vi "FTW-DevUtil-CLFNPrototypes.vi"(0 "VI Ref":refnum<vi>, 11 "error in":errorcluster) -> (4 "VI Ref out":refnum<vi>, 6 "CLFNs":T1[](array[typedef]), 15 "error out":errorcluster)   [LabVIEW 2015]
uses:
  FTW-DevUtil-CLFNPrototype.ctl
panel:
  # "Inputs"
  # "Outputs"
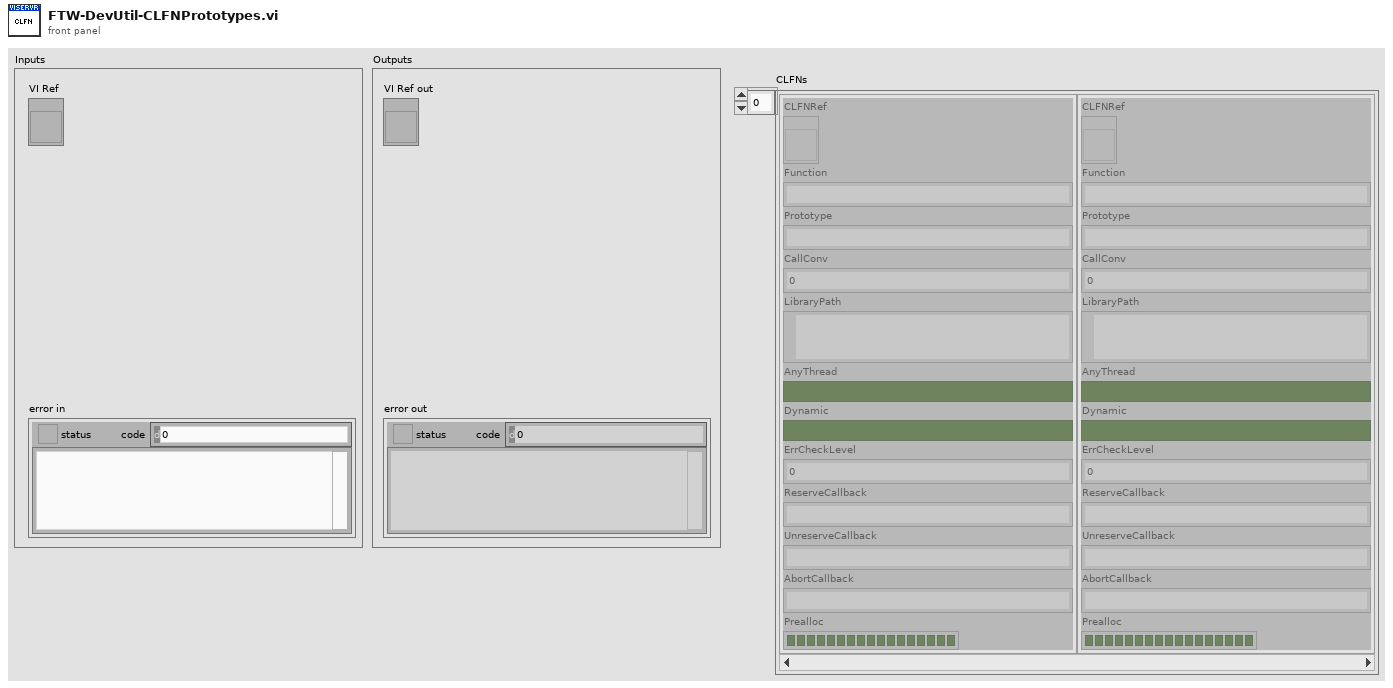
[diagram p1: front panel]
types:
  T1 = typedef "FTW-DevUtil-CLFNPrototype.ctl" = cluster{"CLFNRef":refnum<vi>, "Function":string, "Prototype":string, "CallConv":u32, "LibraryPath":path, "Debug":bool, "Debug":bool, "ErrCheckLevel":u32, "ReserveCallback":string, "UnreserveCallback":string, "AbortCallback":string, "Prealloc":bool[]}
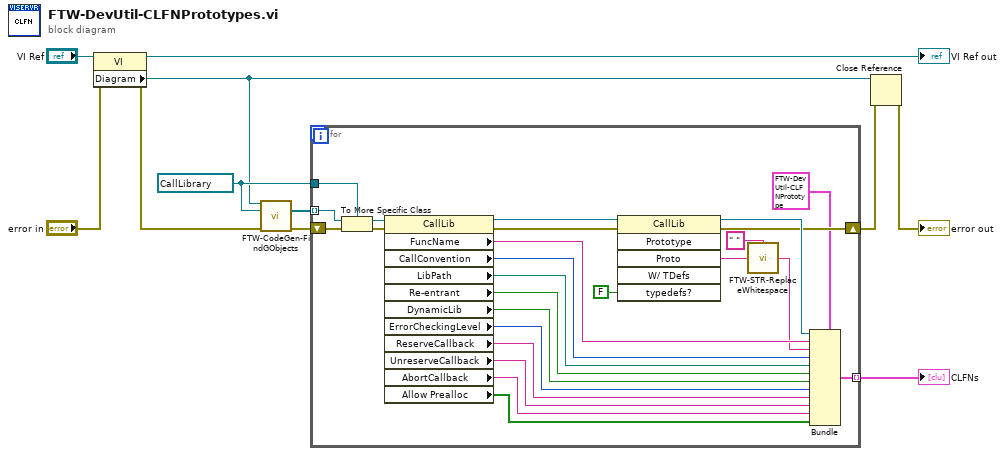
[diagram p0: block diagram]
diagram:
  w9 = refnum<vi> refnum ("GObject")
  n1 = property class="VI"(reference="VI Ref", error in="error in") -> (reference out=→"VI Ref out":refnum<vi>, error out=w4:errorcluster, "Diagram"=w3:refnum<vi>)
  n2 = call "FTW-CodeGen-FindGObjects.vi"("GObject to Traverse"=w3, "Class Type Reference"=w9, "error in"=w4) -> ("GObject Instances"=w11:refnum<vi>[], "error out"=w10:errorcluster)  [unwired: 11 in]
  n3 = for {
    tunnel: w11 -> [w36] mode=indexing
    tunnel: w9 -> [w35]
    tunnel: [w32] -> w7 mode=indexing
    shift-right: [w13] -> w2
    shift-left: w10 -> [w34]
    n4 = To More Specific Class(target class=w35, reference=w36, error in=w34) -> (specific class reference=w20:refnum<vi>, error out=w33:errorcluster)
    n5 = property class="CallLib"(reference=w20, error in=w33) -> (reference out=w23:refnum<vi>, error out=w14:errorcluster, "FuncName"=w16:string, "CallConvention"=w31:u32, "LibPath"=w30:path, "Re-entrant"=w28:bool, "DynamicLib"=w29:bool, "ErrorCheckingLevel"=w27:u32, "ReserveCallback"=w26:string, "UnreserveCallback"=w25:string, "AbortCallback"=w24:string, "Allow Prealloc"=w19:bool[])
    n6 = invoke class="CallLib" method="Prototype"(reference=w23, error in=w14, "typedefs?"=FALSE ("Include Typedefs?")) -> (reference out=w22:refnum<vi>, error out=w13:errorcluster, "Proto"=w18:string)  [unwired: 3 in, 3 out]
    n7 = call "FTW-STR-ReplaceWhitespace.vi"("Replace Spaces With..."=" ", "Input"=w18) -> ("Output"=w15:string)  [unwired: 2 in]
    n8 = Bundle(cluster=T1 {"CLFNRef"=refnum, "Function"="", "Prototype"="", "CallConv"=0, "LibraryPath"=path "", "Debug"=FALSE, "Debug"=FALSE, "ErrCheckLevel"=0, "ReserveCallback"="", "UnreserveCallback"="", "AbortCallback"="", "Prealloc"=[]} ("CLFN"), "CLFNRef"=w22, "Function"=w16, "Prototype"=w15, "CallConv"=w31, "LibraryPath"=w30, "Debug"=w28, "Debug"=w29, "ErrCheckLevel"=w27, "ReserveCallback"=w26, "UnreserveCallback"=w25, "AbortCallback"=w24, "Prealloc"=w19) -> (w32:T1)
  }
  "CLFNs" <- w7
  n9 = Close Reference(reference=w3, error in (no error)=w2) -> (error out=→"error out":errorcluster)
